vi "Panther Dashboard.vi"(8 "error in":errorcluster, 11 "Include Dependencies (T)":bool=TRUE) -> (0 "error out":errorcluster)   [LabVIEW 2020]
uses:
  Panther Dashboard Project/Panter Dashboard/Panter Dashboard.lvlib
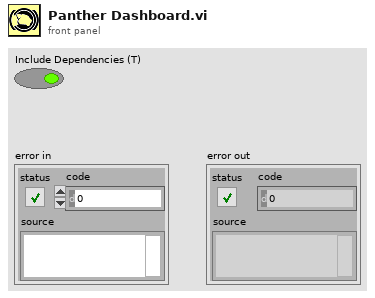
[diagram p1: front panel]
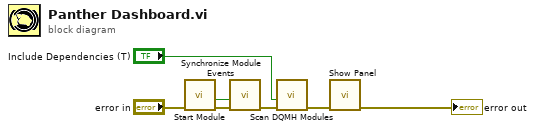
[diagram p0: block diagram]
diagram:
  n1 = call "Start Module.vi"("error in"="error in") -> ("error out"=w7:errorcluster, "Wait for Event Sync?"=w2:bool)  [unwired: 7 in, 2 out]
  n2 = call "Synchronize Module Events.vi"("error in"=w7, "Wait for Event Sync?"=w2) -> ("error out"=w6:errorcluster)  [unwired: 9 in]
  n3 = call "Scan DQMH Modules.vi"("error in"=w6, "Include Dependencies"="Include Dependencies (T)") -> ("error out"=w5:errorcluster)  [unwired: 9 in]
  n4 = call "Show Panel.vi"("error in (no error)"=w5) -> ("error out"=→"error out":errorcluster)  [unwired: 10 in]
